vi "Write Data.vi"(7 "Write Mask":bool[](array[boolean]), 8 "error in (no error)":errorcluster, 9 "Values":dbl[](array[numeric]), 10 "output data access":T1={"Modbus Type"=enum."Input Register", "id"=0, "start"=0, "length"=0, "Channel Data"=[]} {"Channel Data"."Mapping"."VS Reference" format="%.0x"}, 11 "Modbus Master in":refnum<class "Modbus Master.lvclass">=refnum) -> (0 "error out":errorcluster)   [LabVIEW 2021, in "Modbus Master Engine.lvlib"]
uses:
  Modbus Master Engine.lvlib
  Modbus API.lvlibp/API/Master/Modbus Master.lvclass
  Bulk Data Access.ctl
  System Explorer/SubVIs/Modbus Type.ctl
  Shared/Controls/Data Model/Channel.ctl
  <vilib>/NI VeriStand/Custom Device API/Custom Device Channel Type.ctl
  Shared/Controls/Data Model/Mapping.ctl
  Shared/Controls/Data Model/DataType.ctl
  <vilib>/NI VeriStand/Custom Device API/Custom Device Item Ref.ctl
  Shared/Modbus Master Shared.lvlib
  <vilib>/NI VeriStand/Custom Device API/Custom Device API.lvlib
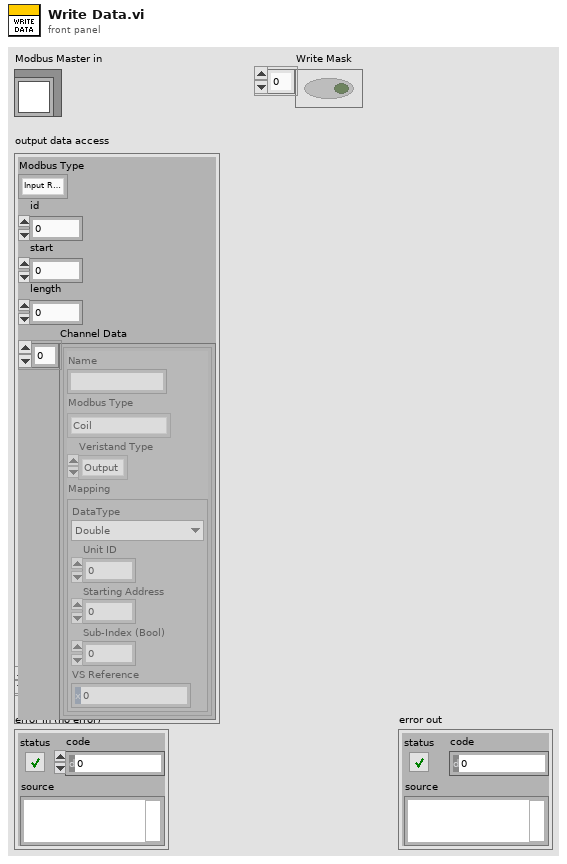
[diagram p1: front panel]
types:
  T1 = typedef "Modbus Master Shared.lvlib/Bulk Data Access.ctl" = cluster{"Modbus Type":T2, "id":u8, "start":u16, "length":u16, "Channel Data":T3[]}
  T2 = typedef "Modbus Master Shared.lvlib/Modbus Type.ctl" = enum16{"Coil", "Discrete Input", "Holding Register", "Input Register"}
  T3 = typedef "Modbus Master Shared.lvlib/Channel.ctl" = cluster{"Name":string, "Modbus Type":T2, "Veristand Type":T4, "Mapping":T5}
  T4 = typedef "Custom Device API.lvlib/Custom Device Channel Type.ctl" = enum16{"Input", "Output"}
  T5 = typedef "Modbus Master Shared.lvlib/Mapping.ctl" = cluster{"DataType":T6, "Unit ID":u8, "Starting Address":u16, "Sub-Index (Bool)":u16, "VS Reference":T7}
  T6 = typedef "Modbus Master Shared.lvlib/DataType.ctl" = enum16{"Double", "Single", "I64", "I32", "I16", "I8", "U64", "U32", "U16", "U8", "Boolean"}
  T7 = typedef "Custom Device API.lvlib/Custom Device Item Ref.ctl" = u64
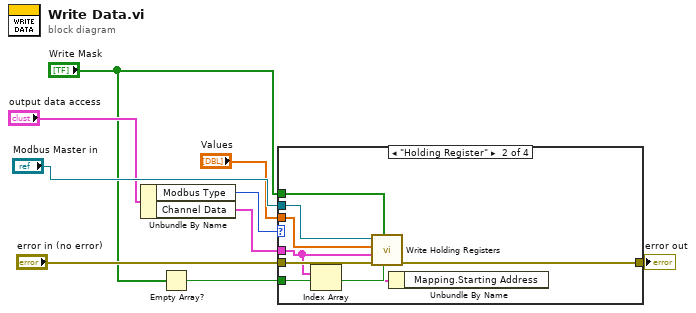
[diagram p0: block diagram]
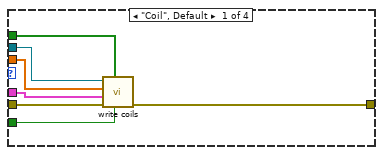
[diagram p2: hidden frame]
diagram:
  n1 = Unbundle By Name("output data access") -> ("Modbus Type"=w4:T2, "Channel Data"=w3:T3[])
  n2 = Empty Array?(array="Write Mask") -> (empty?=w1:bool)
  n3 = case shown="\"Holding Register\"" w4 {
    tunnel: "Modbus Master in" -> [w11 w24 _ _]
    tunnel: [w16 w23 w25 w26] -> w6
    tunnel: "error in (no error)" -> [w15 w22 w25 w26]
    tunnel: w3 -> [w12 w18 _ _]
    tunnel: "Write Mask" -> [w14 w21 _ _]
    tunnel: "Values" -> [w13 w19 _ _]
    tunnel: w1 -> [w10 w20 _ _]
    frame "Coil", Default {
      n4 = call "write coils.vi"("Ignore Mask?"=w10, "Write Mask"=w14, "error in (no error)"=w15, "Channel Data"=w12, "Values"=w13, "Modbus Master in"=w11) -> ("error out"=w16:errorcluster)  [unwired: 5 in]
    }
    frame "Holding Register" {
      n5 = Index Array(array=w18) -> (element=w17:T3)  [unwired: 1 in]
      n6 = call "Write Holding Registers.vi"("Ignore Mask?"=w20, "Regs to Write"=w21, "error in (no error)"=w22, "Channel Data"=w18, "Values"=w19, "Modbus Master in"=w24) -> ("error out"=w23:errorcluster)  [unwired: 5 in]
      n7 = Unbundle By Name(w17) -> ()  [unwired: 1 out]
    }
    frame "Input Register" {
      # "Master can't write\nInput Regs"
    }
    frame "Discrete Input" {
      # "Master can't write\nDiscrete Inputs"
    }
  }
  "error out" <- w6
